vi "P6.vi"() -> ()   [LabVIEW 2019]
uses:
  <vilib>/numeric/Random Number (Range) DBL.vi
panel:
  in  "Stop Button":bool
  out "Resultat":dbl
  in  "Divisible":dbl
  out "Número Aleatori":dbl
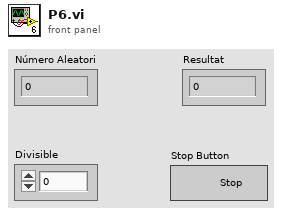
[diagram p1: front panel]
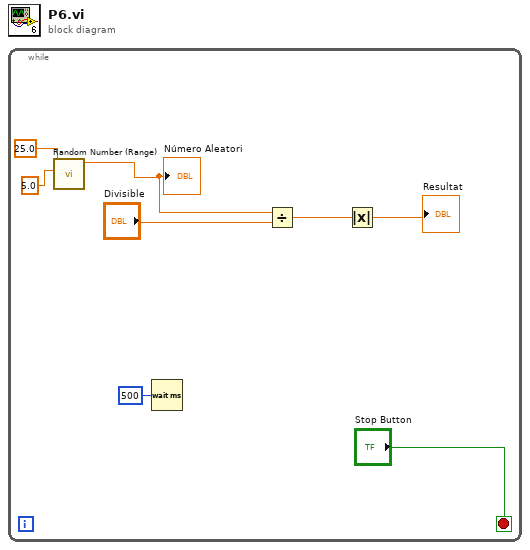
[diagram p0: block diagram]
diagram:
  n1 = while {
    stop <- "Stop Button" stop-if-true
    n2 = call-poly <vilib>:"Random Number (Range).vi"("lower bound (0)"=5.0, "upper bound (100)"=25.0 ("lower bound (0)")) -> ("number"=w7:dbl)  [unwired: 9 in]
    "Número Aleatori" <- w7
    n3 = Wait (ms)(milliseconds to wait=u32 500) -> ()  [unwired: 1 out]
    n4 = Divide(x=w7, y="Divisible") -> (x/y=w5:dbl)
    n5 = Absolute Value(x=w5) -> (abs(x)=→"Resultat":dbl)
  }
